vi "can_speed.vi"(11 "Output Array":string[][](array[string])) -> (0 "v3":u16, 2 "v2":u16, 5 "v 1":u16, 8 "raw":cluster{u16, u16, u16, u16, u16, u16})   [LabVIEW 2015]
panel:
  out "resulting string":string
  out "string":string
  out "element 3":string
  out "v 2":u16
  out "v2 2":u16
  out "v3  2":u16
  out "element 2":string
  out "element":string
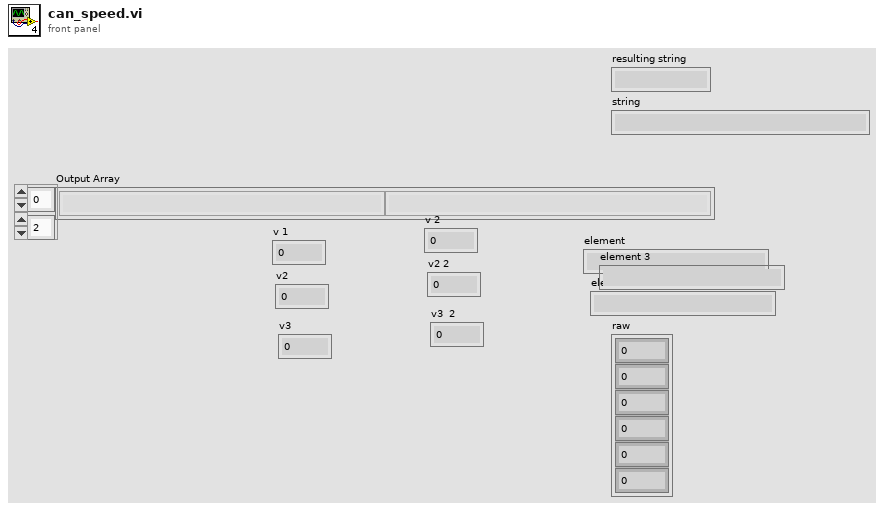
[diagram p1: front panel]
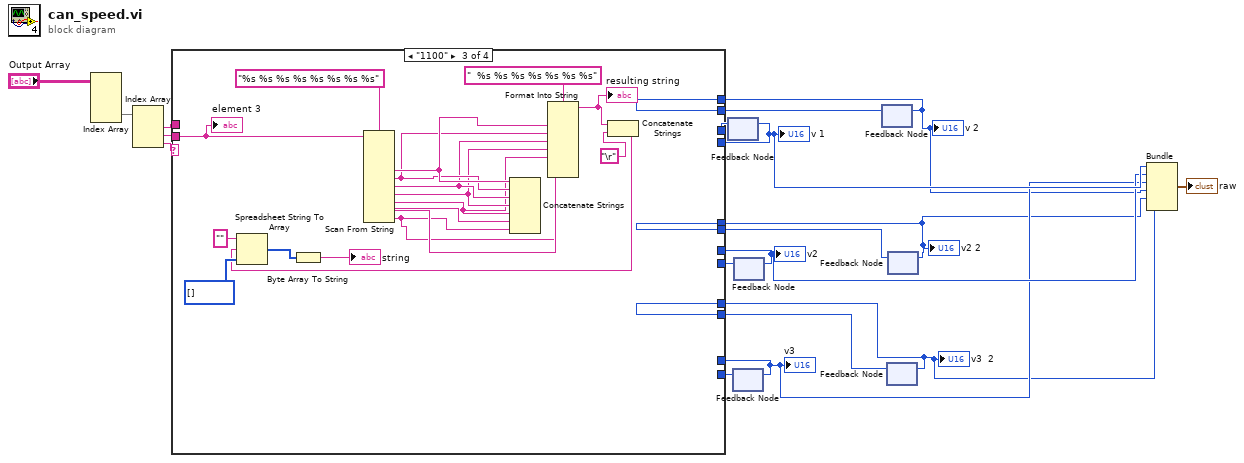
[diagram p0: block diagram]
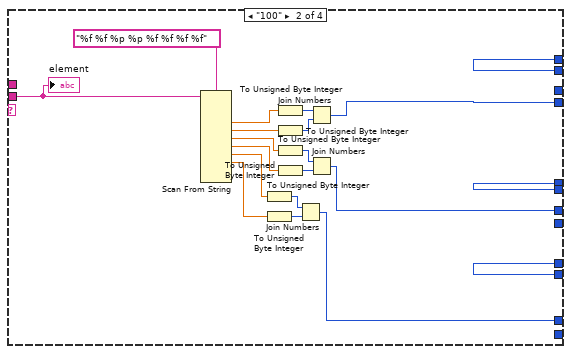
[diagram p3: hidden frame]
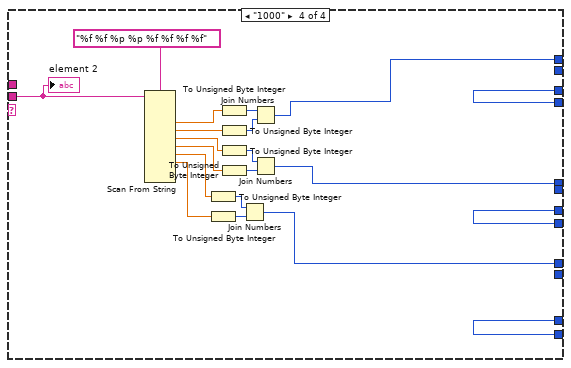
[diagram p4: hidden frame]
diagram:
  n1 = Index Array(array="Output Array") -> (element #2=w17:string[])  [unwired: 4 in, 1 out]
  n2 = Index Array(array=w17) -> (element #1=w12:string, element #2=w16:string, element #3=w15:string)  [unwired: 3 in]
  n3 = feedback #1() -> (w14:u16)  [unwired: 1 in]
  n4 = feedback #2() -> (w11:u16)  [unwired: 1 in]
  n5 = feedback #3() -> (w13:u16)  [unwired: 1 in]
  n6 = feedback #4() -> (w10:u16)  [unwired: 1 in]
  n7 = feedback #5() -> (w8:u16)  [unwired: 1 in]
  n8 = feedback #6() -> (w9:u16)  [unwired: 1 in]
  n9 = case shown="\"1100\"" w15 {
    tunnel: w16 -> [_ w35 w60 w75]
    tunnel: [w24 w28 _ w67] -> w7
    tunnel: [w23 w34 _ w66] -> w6
    tunnel: w14 -> [w24 _ _ w67]
    tunnel: w13 -> [w23 _ _ w66]
    tunnel: w12 -> [_ _ _ _]
    tunnel: [w22 w29 _ w65] -> w5
    tunnel: w11 -> [w22 _ _ w65]
    tunnel: [w21 w27 w63 w70] -> w4
    tunnel: [w20 w26 w62 w69] -> w3
    tunnel: [w19 w25 w61 w68] -> w2
    tunnel: w10 -> [w21 w27 w63 _]
    tunnel: w9 -> [w20 w26 w62 _]
    tunnel: w8 -> [w19 w25 w61 _]
    frame "False", Default {
    }
    frame "100" {
      n10 = Scan From String(format string="%f %f %p %p %f %f %f %f", input string=w35) -> (output 1=w43:dbl, output 2=w42:dbl, output 3=w41:dbl, output 4=w38:dbl, output 5=w31:dbl, output 6=w30:dbl)  [unwired: 12 in, 3 out]
      n11 = To Unsigned Byte Integer(number=w31) -> (unsigned 8bit integer=w32:u8)
      n12 = To Unsigned Byte Integer(number=w30) -> (unsigned 8bit integer=w33:u8)
      n13 = To Unsigned Byte Integer(number=w43) -> (unsigned 8bit integer=w40:u8)
      n14 = To Unsigned Byte Integer(number=w42) -> (unsigned 8bit integer=w39:u8)
      n15 = To Unsigned Byte Integer(number=w41) -> (unsigned 8bit integer=w37:u8)
      n16 = To Unsigned Byte Integer(number=w38) -> (unsigned 8bit integer=w36:u8)
      n17 = Join Numbers(hi=w32, lo=w33) -> ((hi.lo)=w29:u16)
      n18 = Join Numbers(hi=w40, lo=w39) -> ((hi.lo)=w28:u16)
      n19 = Join Numbers(hi=w37, lo=w36) -> ((hi.lo)=w34:u16)
      "element" <- w35
    }
    frame "1100" {
      n20 = Scan From String(format string="%s %s %s %s %s %s %s %s", input string=w60) -> (output 2=w55:string, output 3=w54:string, output 4=w53:string, output 5=w52:string, output 6=w51:string, output 7=w50:string, output 8=w49:string)  [unwired: 11 in, 3 out]
      n21 = Concatenate Strings(w55, w54, w53, w52, w51, w50, w49) -> ()  [unwired: 1 out]
      n22 = Format Into String(format string="  %s %s %s %s %s %s %s", w55, w54, w53, w52, w51, w50, w49) -> (resulting string=w47:string)  [unwired: 2 in, 1 out]
      "resulting string" <- w47
      n23 = Concatenate Strings(w47, "\r") -> (w45:string)
      n24 = Spreadsheet String To Array(format string="", spreadsheet string=w45, array type (2D Dbl)=u8[] [] ("unsigned byte array")) -> (array=w58:u8[])  [unwired: 1 in]
      n25 = Byte Array To String(unsigned byte array=w58) -> (string=→"string":string)
      "element 3" <- w60
    }
    frame "1000" {
      n26 = Scan From String(format string="%f %f %p %p %f %f %f %f", input string=w75) -> (output 1=w83:dbl, output 2=w82:dbl, output 3=w81:dbl, output 4=w78:dbl, output 5=w72:dbl, output 6=w71:dbl)  [unwired: 12 in, 3 out]
      n27 = To Unsigned Byte Integer(number=w72) -> (unsigned 8bit integer=w73:u8)
      n28 = To Unsigned Byte Integer(number=w71) -> (unsigned 8bit integer=w74:u8)
      n29 = To Unsigned Byte Integer(number=w83) -> (unsigned 8bit integer=w80:u8)
      n30 = To Unsigned Byte Integer(number=w82) -> (unsigned 8bit integer=w79:u8)
      n31 = To Unsigned Byte Integer(number=w81) -> (unsigned 8bit integer=w77:u8)
      n32 = To Unsigned Byte Integer(number=w78) -> (unsigned 8bit integer=w76:u8)
      n33 = Join Numbers(hi=w73, lo=w74) -> ((hi.lo)=w68:u16)
      n34 = Join Numbers(hi=w80, lo=w79) -> ((hi.lo)=w70:u16)
      n35 = Join Numbers(hi=w77, lo=w76) -> ((hi.lo)=w69:u16)
      "element 2" <- w75
    }
  }
  "v 1" <- w7
  "v2" <- w6
  "v3" <- w5
  "v 2" <- w4
  "v2 2" <- w3
  "v3  2" <- w2
  n36 = feedback-in #1(w7) -> ()
  n37 = feedback-in #2(w5) -> ()
  n38 = feedback-in #3(w6) -> ()
  n39 = feedback-in #4(w4) -> ()
  n40 = feedback-in #5(w2) -> ()
  n41 = feedback-in #6(w3) -> ()
  n42 = Bundle(w7, w6, w5, w4, w3, w2) -> (→"raw":cluster{u16, u16, u16, u16, u16, u16})  [unwired: 1 in]
